vi "SubVI_PulseOnRise_Teleop.vi"(1 "Input":bool, 2 "Number of milliseconds to wait.\n~20ms precision.":i32=12) -> (0 "RisingPulse":bool)   [LabVIEW 2017]
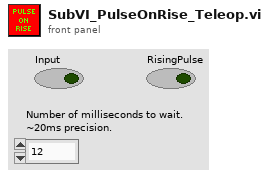
[diagram p1: front panel]
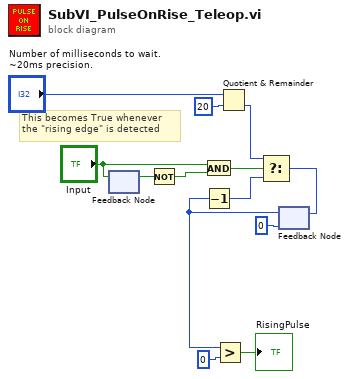
[diagram p0: block diagram]
diagram:
  # "This becomes True whenever \nthe \"rising edge\" is detected"
  n1 = feedback #1() -> (w6:bool)  [unwired: 1 in]
  n2 = feedback-in #1("Input") -> ()
  n3 = Not(x=w6) -> (.not. x?=w7:bool)
  n4 = And(x="Input", y=w7) -> (x .and. y?=w4:bool)
  n5 = Quotient & Remainder(x="Number of milliseconds to wait.\n~20ms precision.", y=20) -> (floor(x/y)=w8:i32)  [unwired: 1 out]
  n6 = feedback #2(0 ("Number of loops to wait \nbetween each change.")) -> (w3:i32)
  n7 = Decrement(x=w3) -> (x-1=w11:i32)
  n8 = Greater?(x=w3, y=0 ("x")) -> (0:→"RisingPulse":bool)
  n9 = Select(t=w8, s=w4, f=w11) -> (s? t:f=w12:i32)
  n10 = feedback-in #2(w12) -> ()
